vi "GF_FireCounterSignal.vi"(1 "DAQmx Global Channel":refnum<k21>="USB_TurnOffBProbeRelay_P0_4") -> (0 "error out":errorcluster)   [LabVIEW 2009]
uses:
  <vilib>/DAQmx/write.llb/DAQmx Write (Counter Time 1Chan 1Samp).vi
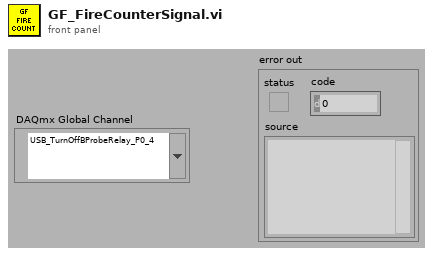
[diagram p1: front panel]
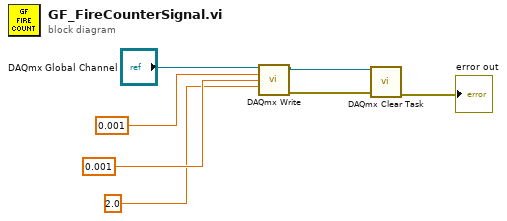
[diagram p0: block diagram]
diagram:
  n1 = call-poly <vilib>:"DAQmx Write.vi"("task/channels in"="DAQmx Global Channel", "high time"=0.001, "low time"=0.001, "timeout"=2.0) -> ("task out"=w1:refnum<k21>, "error out"=w2:errorcluster)  [unwired: 9 in, 1 out]
  n2 = call <vilib>:"DAQmx Clear Task.vi"("task in"=w1, "error in"=w2) -> ("error out"=→"error out":errorcluster)  [unwired: 13 in]
